vi "waveform1.vi"() -> ()   [LabVIEW 2021]
panel:
  out "Waveform Graph":waveform(dbl)(graph)
  in  "Waveform":waveform(dbl)
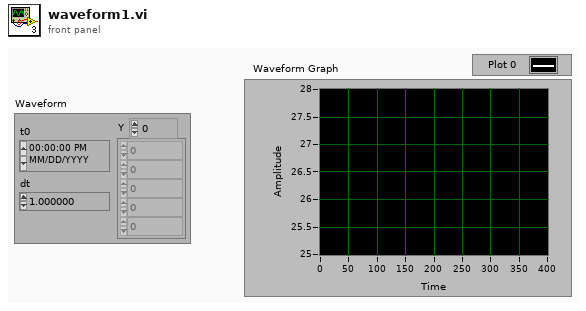
[diagram p1: front panel]
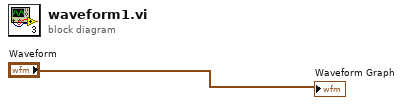
[diagram p0: block diagram]
diagram:
  "Waveform Graph" <- "Waveform"
